vi "Keithley24xx_Read.vi"(3 "error in (no error)":errorcluster, 4 "Function (0: Volts)":u16(ring) items=["Volts", "Current", "Resistance"], 5 "VISA resource name":refnum<visa-resource-name>) -> (0 "error out":errorcluster, 1 "Out":sgl, 2 "VISA resource name out":refnum<visa-resource-name>)   [LabVIEW 2014]
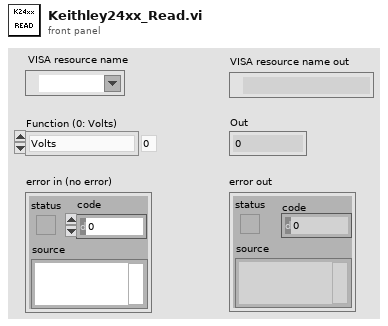
[diagram p1: front panel]
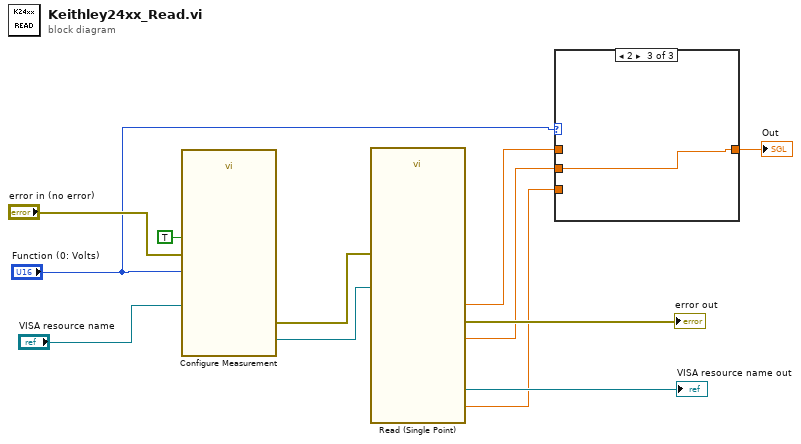
[diagram p0: block diagram]
diagram:
  n1 = call "Configure Measurement.vi"("error in (no error)"="error in (no error)", "Enable Auto Range (T:Enable)"=TRUE, "Function (0: Volts)"="Function (0: Volts)", "VISA resource name"="VISA resource name") -> ("error out"=w10:errorcluster, "VISA resource name out"=w11:refnum<visa-resource-name>)  [unwired: 6 in]
  n2 = call "Read (Single Point).vi"("VISA resource name"=w11, "error in (no error)"=w10) -> ("Voltage"=w4:sgl, "VISA resource name out"=→"VISA resource name out":refnum<visa-resource-name>, "Current"=w2:sgl, "Resistance"=w1:sgl, "error out"=→"error out":errorcluster)  [unwired: 7 in, 2 out]
  n3 = case shown="2" "Function (0: Volts)" {
    tunnel: w4 -> [w13 _ _]
    tunnel: [w13 w14 w15] -> w3
    tunnel: w2 -> [_ w14 _]
    tunnel: w1 -> [_ _ w15]
    frame 0, Default {
    }
    frame 1 {
    }
    frame 2 {
    }
  }
  "Out" <- w3
